vi "CC Script Parse Random Dither.vi"(8 "error in (no error)":errorcluster, 9 "To String?":bool=TRUE, 10 "Dithering in":T1={"Count"=1, "Radius"=1.0, "Name"=""}, 11 "Dither Parameters":string="\"Rnadome Dither Mispeller\" Count=3,Radius=1.23") -> (0 "error out":errorcluster, 2 "Dithering out":T1={"Count"=1, "Radius"=1.0, "Name"=""}, 3 "resulting string":string)   [LabVIEW 2021]
uses:
  typedefs/CC cluster Random Dithering.ctl
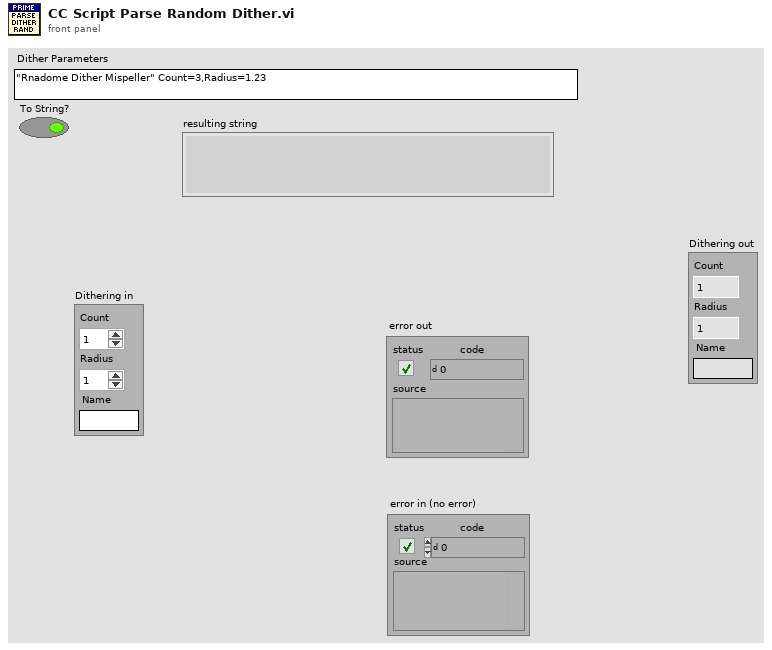
[diagram p1: front panel]
types:
  T1 = typedef "CC cluster Random Dithering.ctl" = cluster{"Count":i32, "Radius":dbl, "Name":string}
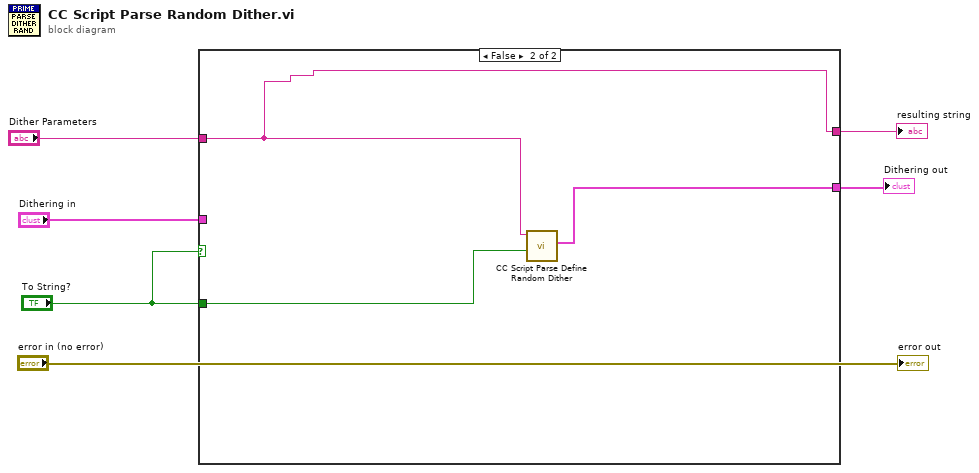
[diagram p0: block diagram]
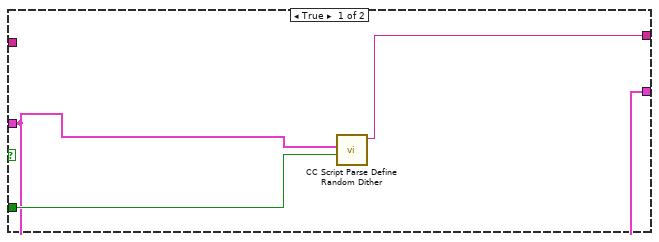
[diagram p2: hidden frame]
diagram:
  n1 = case shown="False" "To String?" {
    tunnel: "Dithering in" -> [w8 _]
    tunnel: [w7 w11] -> w4
    tunnel: "Dither Parameters" -> [_ w11]
    tunnel: "To String?" -> [w9 w12]
    tunnel: [w8 w10] -> w1
    frame True {
      n2 = call "CC Script Parse Define Random Dither.vi"("To String?"=w9, "Random Dither in"=w8) -> ("Script String out"=w7:string)  [unwired: 7 in, 2 out]
    }
    frame False {
      n3 = call "CC Script Parse Define Random Dither.vi"("To String?"=w12, "Dither Parameters"=w11) -> ("Random Dither out"=w10:T1)  [unwired: 7 in, 2 out]
    }
  }
  "resulting string" <- w4
  "Dithering out" <- w1
  "error out" <- "error in (no error)"
